vi "写入被运算数字符.vi"(8 "error in (no error)":errorcluster caption="错误输入（无错误）", 10 "被运算数字符":string, 11 "计算器类输入":refnum<class "计算器类.lvclass">) -> (0 "error out":errorcluster caption="错误输出", 3 "计算器类输出":refnum<class "计算器类.lvclass">)   [LabVIEW 2020, in "计算器类.lvclass"]
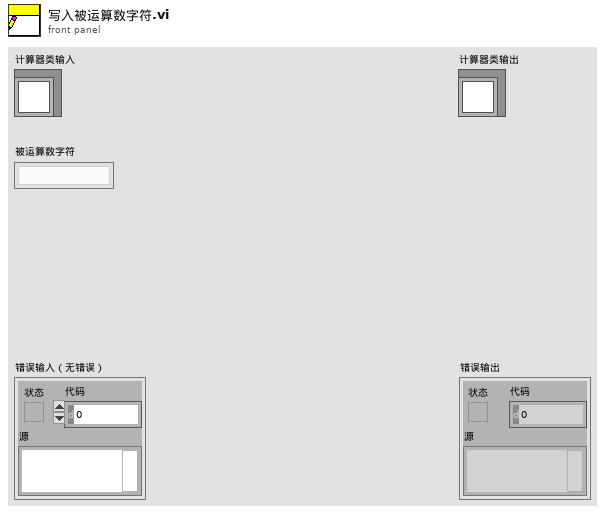
[diagram p1: front panel]
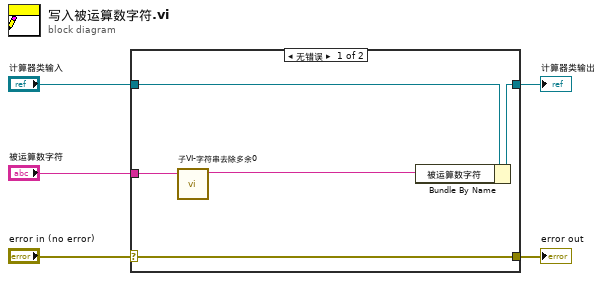
[diagram p0: block diagram]
diagram:
  n1 = case shown="无错误" "error in (no error)" {
    selector: "error in (no error)" -> [w10 w11]
    tunnel: [w10 w11] -> w4
    tunnel: [w8 w12] -> w2
    tunnel: "计算器类输入" -> [w9 w12]
    tunnel: "被运算数字符" -> [w7 _]
    frame No Error {
      n2 = call "子VI-字符串去除多余0.vi"("带0字符串"=w7) -> ("result string"=w6:string)  [unwired: 10 in]
      n3 = Bundle By Name(cluster=w9, "被运算数字符"=w6) -> (w8:refnum<class "计算器类.lvclass">)
    }
    frame Error {
    }
  }
  "error out" <- w4
  "计算器类输出" <- w2
